vi "TimeString2Time24.vi"(10 "Time Stamp":timestamp, 11 "時間字串":string) -> (2 "時間字串":string, 3 "date/time string":string)   [LabVIEW 2019]
uses:
  <vilib>/addons/database/Auxilliary.llb/DB Tools Format Datetime String (Time Stamp).vi
  <vilib>/addons/database/NI_Database_API.lvlib
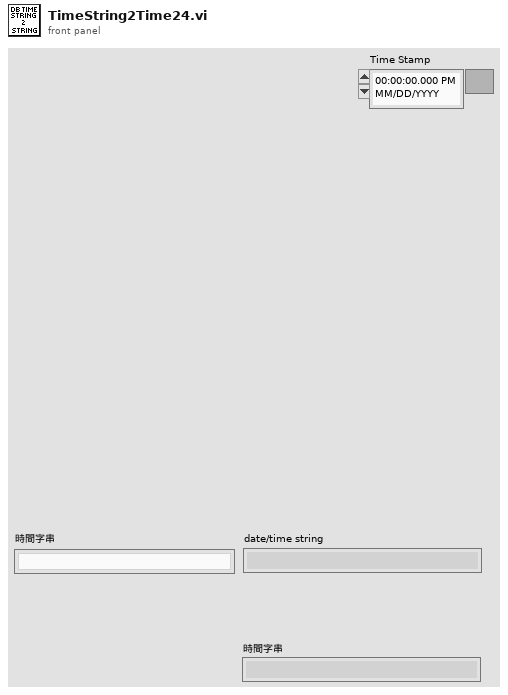
[diagram p1: front panel]
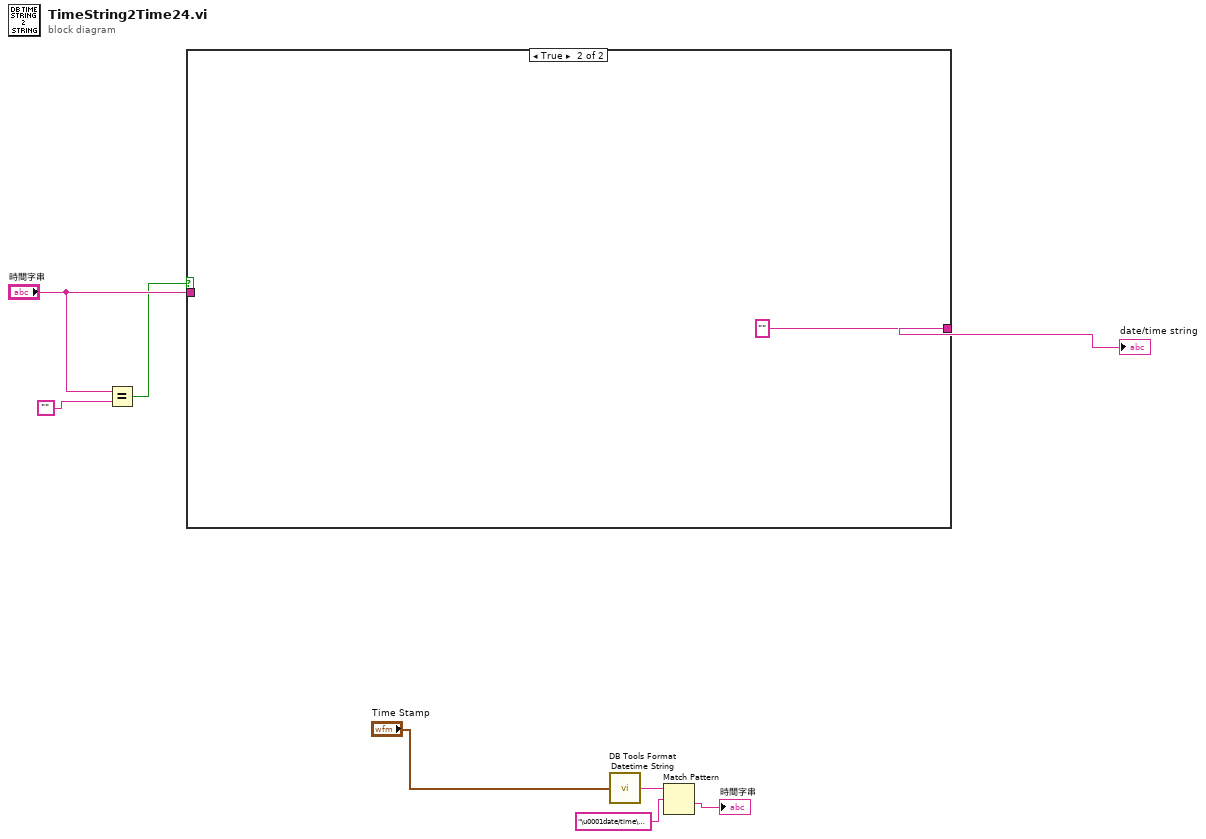
[diagram p0: block diagram]
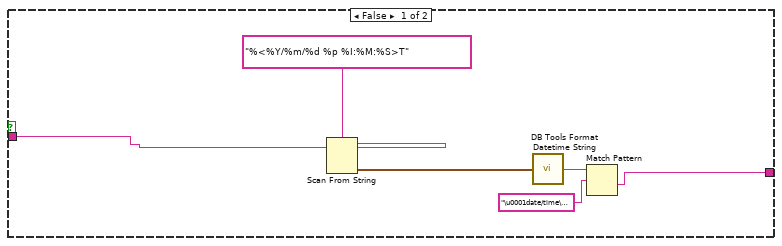
[diagram p2: hidden frame]
diagram:
  n1 = Equal?(x="時間字串", y="") -> (x = y?=w6:bool)
  n2 = case shown="True" w6 {
    tunnel: "時間字串" -> [w13 _]
    tunnel: [w9 "" ("date/time string")] -> w1
    frame False {
      n3 = Scan From String(format string="%<%Y/%m/%d %p %I:%M:%S>T", input string=w13) -> (output 1=w10:timestamp)  [unwired: 3 in, 3 out]
      n4 = call-poly <vilib>:"DB Tools Format Datetime String.vi"("time stamp"=w10) -> ("date/time string"=w11:string)
      n5 = Match Pattern(string=w11, regular expression="\u0001date/time\u0001" ("search string")) -> (after substring=w9:string)  [unwired: 1 in, 3 out]
    }
    frame True {
    }
  }
  "date/time string" <- w1
  n6 = call-poly <vilib>:"DB Tools Format Datetime String.vi"("time stamp"="Time Stamp") -> ("date/time string"=w3:string)
  n7 = Match Pattern(string=w3, regular expression="\u0001date/time\u0001" ("search string")) -> (after substring=→"時間字串":string)  [unwired: 1 in, 3 out]
